vi "Plugin GUID.vi"() -> (3 "GUID":string="88fcfa75-3196-4ae9-a459-f2e46a72afc7")   [LabVIEW 2017, in "Data Sharing Framework System Explorer.lvlib"]
uses:
  Data Sharing Framework System Explorer.lvlib
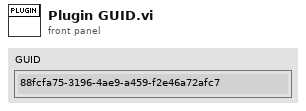
[diagram p1: front panel]
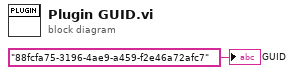
[diagram p0: block diagram]
diagram:
  "GUID" <- "88fcfa75-3196-4ae9-a459-f2e46a72afc7" ("Data Sharing Framework")
